vi "DLaserpowerEOM.vi"(2 "error in (no error)":errorcluster) -> (0 "error out":errorcluster)   [LabVIEW 2011]
uses:
  <vilib>/DAQmx/write.llb/DAQmx Write (Analog DBL 1Chan 1Samp).vi
  <vilib>/DAQmx/read.llb/DAQmx Read (Analog DBL 1Chan 1Samp).vi
  <vilib>/DAQmx/create/channels.llb/DAQmx Create Channel (AO-Voltage-Basic).vi
  <vilib>/DAQmx/create/channels.llb/DAQmx Create Channel (AI-Voltage-Basic).vi
  <vilib>/DAQmx/miscellaneous.llb/DAQmx Fill In Error Info.vi
  <vilib>/gmath/NI_Gmath.lvlib
  <vilib>/Analysis/NI_AALPro.lvlib
panel:
  out "DiodeUeff":dbl
  out "interpolation W/V":dbl format="%0.2f"
  in  "W/V":dbl[](array[numeric])=[1.0, 2.0, 1.0]
  in  "nm":dbl[](array[numeric])=[700.0, 900.0, 1100.0]
  out "value out":string
  out "Laserpower":dbl
  out "Transmission at EOM":dbl
  out "Voltage-out":dbl format="%0.2f"
  out "Total transmission":dbl
  out "Waveform Chart":cluster{"mW to serach":dbl, dbl}(graph)
  out "Found W":dbl=27.59081560595219
  out "nm":dbl=751.0
  out "set Power in W":dbl=26.516448089513062
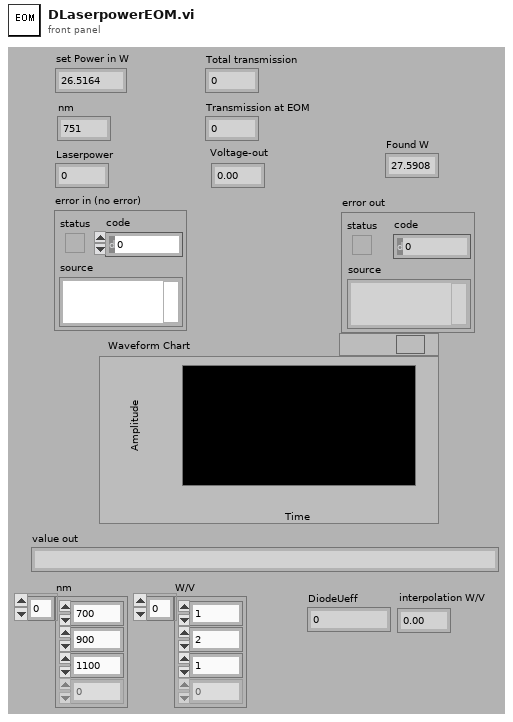
[diagram p1: front panel]
types:
  T1 = enum16{"None/#Datasets", "Clear", "TagValueOf#", "AddValues", "ReadValue", "ChangeValue", "Get all"}
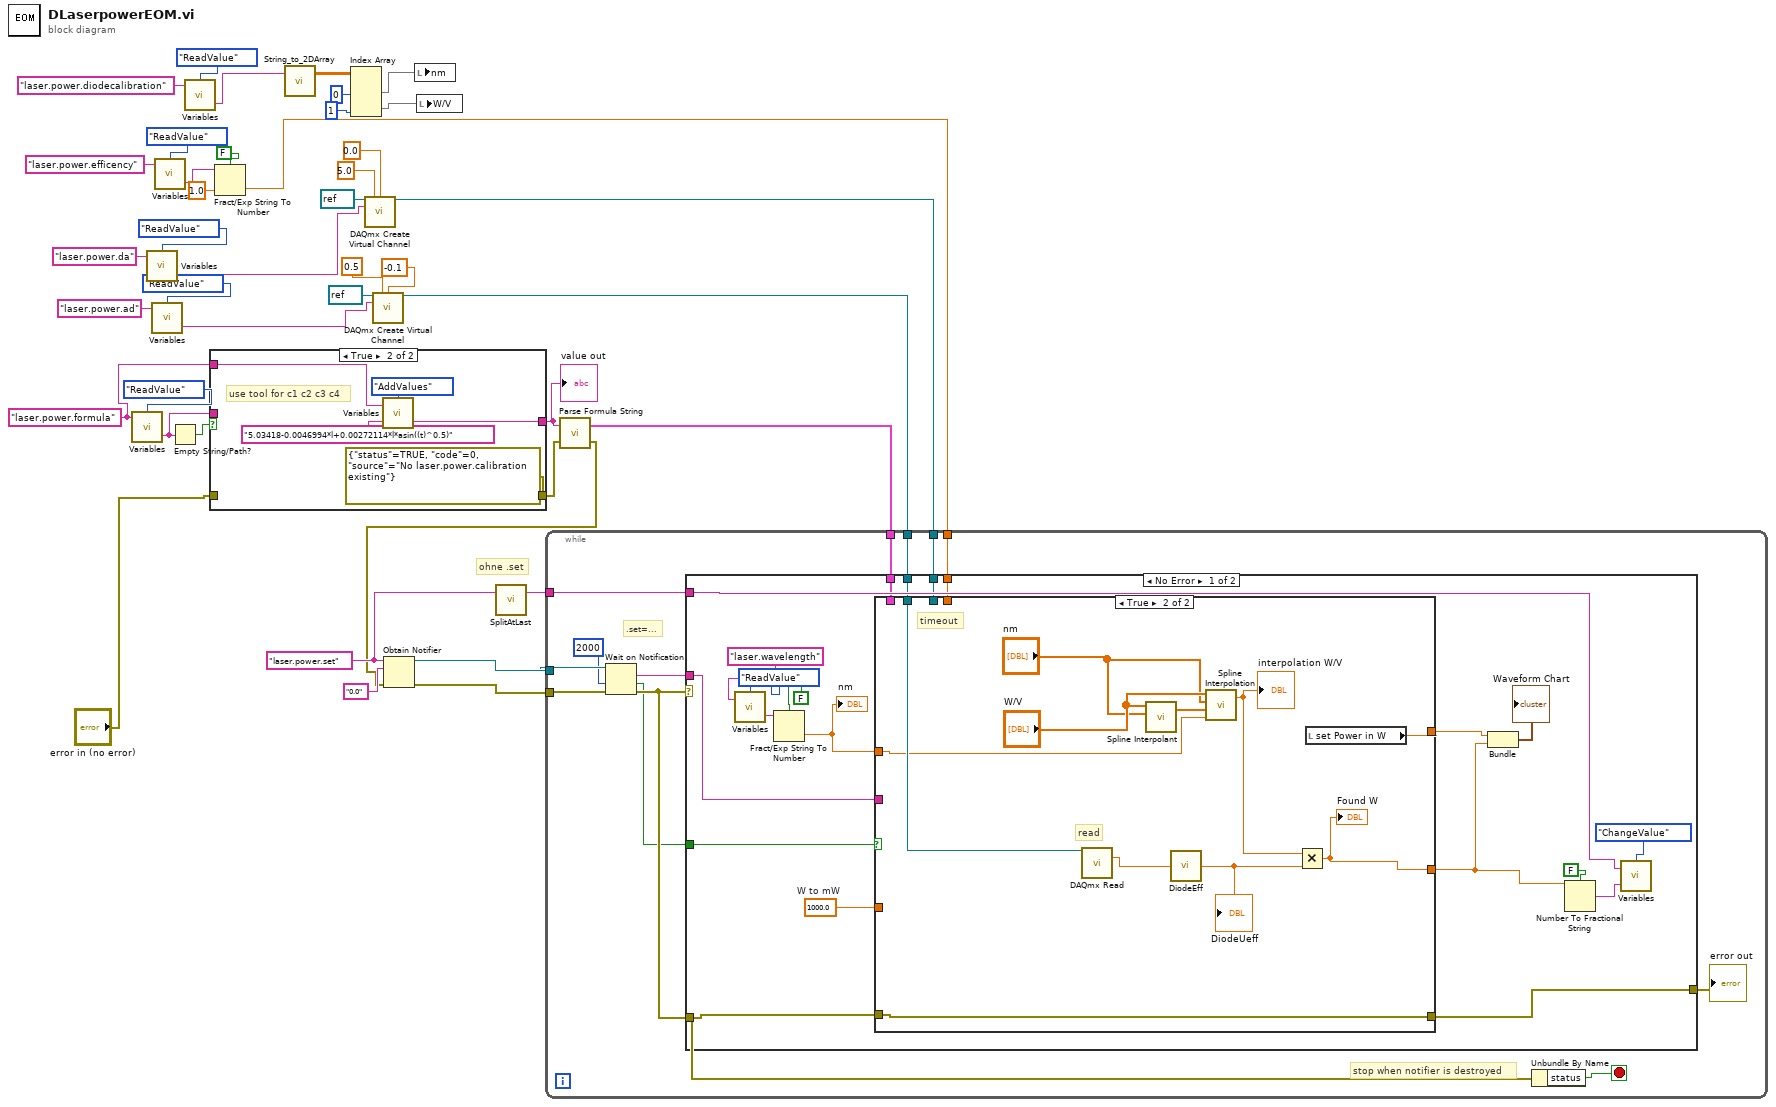
[diagram p0: block diagram]
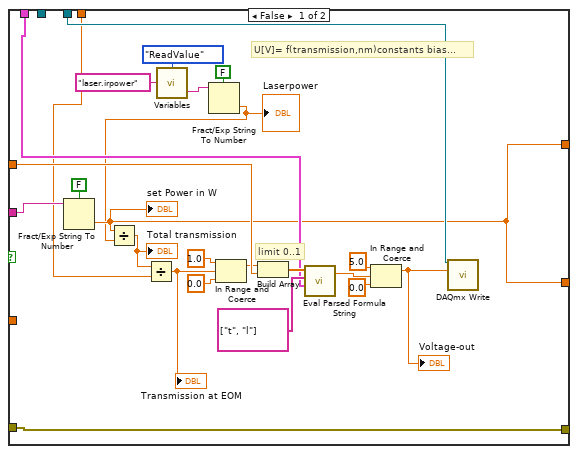
[diagram p3: hidden frame]
diagram:
  w9 = "laser.power.formula" ("Tag in")
  w39 = "laser.power.set" ("name (unnamed)")
  # "ohne .set"
  n1 = call "Variables.vi"("Tag in"=w9, "Command"=T1."ReadValue") -> ("value out"=w10:string)  [unwired: 1 in, 2 out]
  n2 = call "Variables.vi"("Tag in"="laser.power.da", "Command"=T1."ReadValue") -> ("value out"=w29:string)  [unwired: 1 in, 2 out]
  n3 = call "Variables.vi"("Tag in"="laser.power.ad", "Command"=T1."ReadValue") -> ("value out"=w28:string)  [unwired: 1 in, 2 out]
  n4 = call "Variables.vi"("Tag in"="laser.power.efficency", "Command"=T1."ReadValue") -> ("value out"=w17:string)  [unwired: 1 in, 2 out]
  n5 = Empty String/Path?(string/path=w10) -> (empty?=w36:bool)
  n6 = call "Variables.vi"("Tag in"="laser.power.diodecalibration", "Command"=T1."ReadValue") -> ("value out"=w6:string)  [unwired: 1 in, 2 out]
  n7 = case shown="True" w36 {
    tunnel: w10 -> [w43 _]
    tunnel: "error in (no error)" -> [w44 _]
    tunnel: [w44 errorcluster {"status"=TRUE, "code"=0, "source"="No laser.power.calibration existing"} ("error in (no error)")] -> w12
    tunnel: [w43 w46] -> w21
    tunnel: w9 -> [_ w45]
    frame False {
      # "Calibration existing"
    }
    frame True {
      # "use tool for c1 c2 c3 c4"
      n8 = call "Variables.vi"("value"="5.03418-0.0046994*l+0.00272114*l*asin((t)^0.5)" ("data do not use \"=\" but \":\""), "Tag in"=w45, "Command"=T1."AddValues") -> ("value out"=w46:string)  [unwired: 2 out]
    }
  }
  "value out" <- w21
  n9 = Fract/Exp String To Number(use system decimal point (T)=FALSE, string=w17, default (0 dbl)=1.0 ("default (0 DBL)")) -> (number=w14:dbl)  [unwired: 1 in, 1 out]
  n10 = call "String_to_2DArray.vi"("String"=w6) -> ("Array"=w5:dbl[][])  [unwired: 3 in, 1 out]
  n11 = Index Array(array=w5, index (col) #1=0 ("disabled index (col)"), index (col) #2=1 ("index (row)")) -> (element #1=w4:dbl[], element #2=w3:dbl[])  [unwired: 2 in]
  n12 = call-poly <vilib>:"DAQmx Create Virtual Channel.vi"("task in"=refnum<k21> refnum, "maximum value"=5.0, "minimum value"=0.0, "physical channels"=w29) -> ("task out"=w22:refnum<k21>)  [unwired: 5 in, 6 out]
  n13 = call-poly <vilib>:"DAQmx Create Virtual Channel.vi"("task in"=refnum<k21> refnum, "maximum value"=0.5, "minimum value"=-0.1, "physical channels"=w28) -> ("task out"=w23:refnum<k21>)  [unwired: 5 in, 6 out]
  n14 = local write "nm"(w4) -> ()
  n15 = local write "W/V"(w3) -> ()
  n16 = call "SplitAtLast.vi"("In-String"=w39) -> ("Front (default)"=w38:string)  [unwired: 1 in, 1 out]
  n17 = call <vilib>:"Parse Formula String.vi"("error in (no error)"=w12, "formula"=w21) -> ("error out"=w11:errorcluster, "Parsed Formula"=w20:cluster{"Table":i32[][], "Y Values":dbl[]})
  n18 = Obtain Notifier(name (unnamed)=w39, notification data type="0.0", error in (no error)=w11) -> (notifier out=w41:refnum<notifier>, error out=w40:errorcluster)  [unwired: 1 in, 1 out]
  n19 = while {
    tunnel: w41 -> [w61]
    tunnel: w40 -> [w60]
    tunnel: w38 -> [w54]
    tunnel: w23 -> [w53]
    tunnel: w22 -> [w52]
    tunnel: w20 -> [w51]
    tunnel: w14 -> [w50]
    stop <- w57 stop-if-true
    # "stop when notifier is destroyed"
    # ".set=..."
    n20 = Wait on Notification(notifier=w61, timeout in ms (-1)=2000, error in (no error)=w60) -> (notification=w59:string, timed out?=w56:bool, error out=w58:errorcluster)  [unwired: 2 out]
    n21 = case shown="No Error" w58 {
      tunnel: [w68 w119] -> w62
      tunnel: w58 -> [w69 w119]
      tunnel: w59 -> [w74 _]
      tunnel: w56 -> [w75 _]
      tunnel: w54 -> [w73 _]
      tunnel: w53 -> [w71 _]
      tunnel: w52 -> [w70 _]
      tunnel: w51 -> [w65 _]
      tunnel: w50 -> [w64 _]
      frame No Error {
        w66 = 1000.0  # W to mW
        n22 = call "Variables.vi"("Tag in"="laser.wavelength", "Command"=T1."ReadValue") -> ("value out"=w81:string)  [unwired: 1 in, 2 out]
        n23 = Fract/Exp String To Number(use system decimal point (T)=FALSE, string=w81) -> (number=w80:dbl)  [unwired: 3 out]
        "nm" <- w80
        n24 = case shown="True" w75 {
          tunnel: [w85 w108] -> w63
          tunnel: w80 -> [w96 w112]
          tunnel: [w98 w115] -> w68
          tunnel: w74 -> [w102 _]
          tunnel: [w85 w117] -> w72
          tunnel: w71 -> [_ w116]
          tunnel: w70 -> [w99 _]
          tunnel: w69 -> [w98 w115]
          tunnel: w66 -> [_ _]
          tunnel: w65 -> [w93 _]
          tunnel: w64 -> [w87 _]
          frame False {
            # "limit 0..1"
            # "U[V]= f(transmission,nm)constants bias..."
            n25 = Fract/Exp String To Number(use system decimal point (T)=FALSE, string=w102) -> (number=w85:dbl)  [unwired: 3 out]
            "set Power in W" <- w85
            n26 = call "Variables.vi"("Tag in"="laser.irpower", "Command"=T1."ReadValue") -> ("value out"=w103:string)  [unwired: 1 in, 2 out]
            n27 = Fract/Exp String To Number(use system decimal point (T)=FALSE, string=w103) -> (number=w84:dbl)  [unwired: 3 out]
            "Laserpower" <- w84
            n28 = Divide ("Transmission")(x=w85, y=w84) -> (x/y=w90:dbl)
            "Total transmission" <- w90
            n29 = Divide(x=w90, y=w87) -> (x/y=w88:dbl)
            "Transmission at EOM" <- w88
            n30 = In Range and Coerce(upper limit=1.0, x=w88, lower limit=0.0) -> (coerced(x)=w89:dbl)  [unwired: 1 out]
            n31 = Build Array(w89, w96) -> (w95:dbl[])
            n32 = call <vilib>:"Eval Parsed Formula String.vi"("Parsed Formula"=w93, "Variables"=string[] ["t", "l"], "X Values"=w95) -> ("y value"=w94:dbl)  [unwired: 1 in, 1 out]
            n33 = In Range and Coerce(upper limit=5.0, x=w94, lower limit=0.0) -> (coerced(x)=w86:dbl)  [unwired: 1 out]
            "Voltage-out" <- w86
            n34 = call-poly <vilib>:"DAQmx Write.vi"("task/channels in"=w99, "data"=w86) -> ()  [unwired: 2 in, 12 out]
          }
          frame True {
            # "timeout"
            # "read"
            n35 = call-poly <vilib>:"DAQmx Read.vi"("task/channels in"=w116) -> ("data"=w118:dbl)  [unwired: 1 in, 13 out]
            n36 = call <vilib>:"Spline Interpolant.vi"("X"="nm", "Y"="W/V") -> ("Interpolant"=w113:dbl[])  [unwired: 2 in, 1 out]
            n37 = call "DiodeEff.vi"("DiodeU"=w118) -> ("DiodeUeff"=w114:dbl)
            "DiodeUeff" <- w114
            n38 = call <vilib>:"Spline Interpolation.vi"("x value"=w112, "Interpolant"=w113, "X"="nm", "Y"="W/V") -> ("interpolation value"=w111:dbl)  [unwired: 1 out]
            "interpolation W/V" <- w111
            n39 = Multiply(x=w111, y=w114) -> (x*y=w108:dbl)
            "Found W" <- w108
            n40 = local read "set Power in W"() -> (w117:dbl)
          }
        }
        n41 = Bundle("set Power in W"=w72, w63) -> (→"Waveform Chart":cluster{"set Power in W":dbl, dbl})  [unwired: 1 in]
        n42 = Number To Fractional String(use system decimal point (T)=FALSE, number=w63) -> (F-format string=w77:string)  [unwired: 2 out]
        n43 = call "Variables.vi"("value"=w77, "Tag in"=w73, "Command"=T1."ChangeValue") -> ()  [unwired: 3 out]
      }
      frame Error {
      }
    }
    "error out" <- w62
    n44 = Unbundle By Name(w58) -> ("status"=w57:bool)
  }
